vi "Interpret Device State.vi"(8 "Error In":errorcluster, 11 "Data In":u8[](array[numeric])) -> (0 "Error Out":errorcluster, 1 "ADS Error Number":u32, 2 "Device State":u16, 3 "ADS State":T1)   [LabVIEW 2016, in "TwinCAT ADS.lvlib"]
uses:
  TwinCAT ADS.lvlib
  TypeDefs/ADS States.ctl
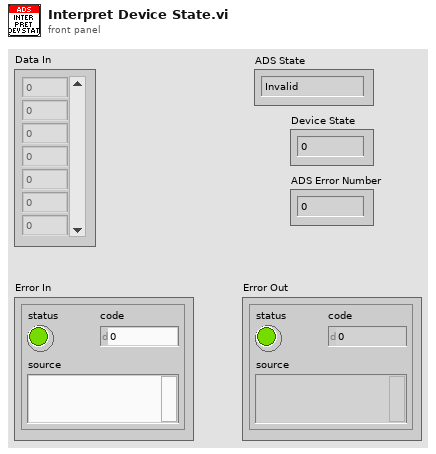
[diagram p1: front panel]
types:
  T1 = typedef "TwinCAT ADS.lvlib/ADS States.ctl" = enum16{"Invalid", "Idle", "Reset", "Init", "Start", "Run", "Stop", "SaveCfg", "LoadCfg", "PowerFailure", "PowerGood", "Error", "Shutdown", "Suspend", "Resume", "Config", "Reconfig"}
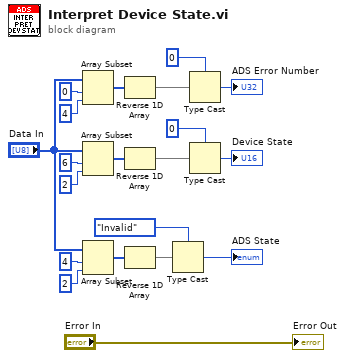
[diagram p0: block diagram]
diagram:
  n1 = Array Subset(array="Data In", index=0, length=4) -> (w20:u8[])
  n2 = Array Subset(array="Data In", index=6, length=2) -> (w6:u8[])
  n3 = Array Subset(array="Data In", index=4, length=2) -> (w13:u8[])
  n4 = Reverse 1D Array(array=w20) -> (reversed array=w17:u8[])
  n5 = Reverse 1D Array(array=w6) -> (reversed array=w2:u8[])
  n6 = Reverse 1D Array(array=w13) -> (reversed array=w12:u8[])
  n7 = Type Cast(type=ADS_States."Invalid", x=w12) -> (*(type *) &x=→"ADS State":T1)
  n8 = Type Cast(type=u32 0, x=w17) -> (*(type *) &x=→"ADS Error Number":u32)
  n9 = Type Cast(type=u16 0, x=w2) -> (*(type *) &x=→"Device State":u16)
  "Error Out" <- "Error In"
